vi "Untitled 7 (SubVI).vi"(8 "y 2":i32, 9 "x 2":i32, 10 "y 1":i32, 11 "x 1":i32) -> (1 "Boolean":bool, 2 "Array":cluster{"x 1":i32, i32}[](array[cluster]))   [LabVIEW 2017]
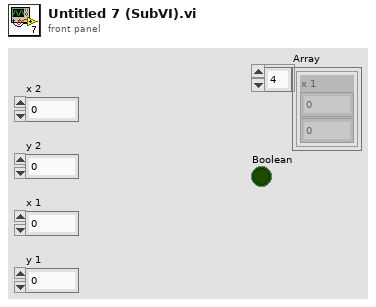
[diagram p1: front panel]
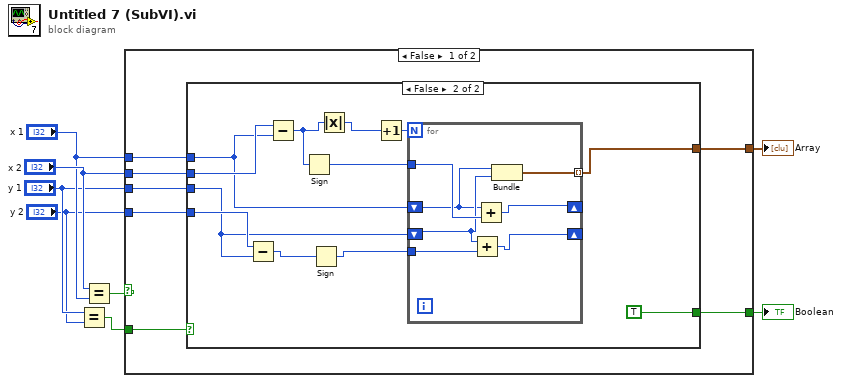
[diagram p0: block diagram]
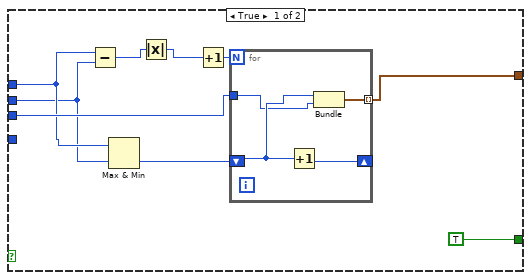
[diagram p2: hidden frame]
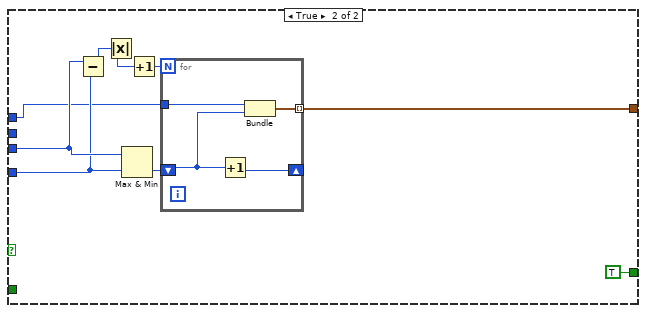
[diagram p3: hidden frame]
diagram:
  n1 = Equal?(x="y 1", y="y 2") -> (x = y?=w7:bool)
  n2 = Equal?(x="x 2", y="x 1") -> (x = y?=w8:bool)
  n3 = case shown="False" w8 {
    tunnel: w7 -> [w15 _]
    tunnel: "x 2" -> [w14 _]
    tunnel: "x 1" -> [w13 w52]
    tunnel: "y 1" -> [w12 w55]
    tunnel: "y 2" -> [w11 w54]
    tunnel: [w10 w51] -> w2
    tunnel: [w9 TRUE] -> w1
    frame False {
      n4 = case shown="False" w15 {
        tunnel: w14 -> [w19 w38]
        tunnel: w13 -> [w20 w35]
        tunnel: w12 -> [w21 w29]
        tunnel: w11 -> [_ w32]
        tunnel: [w22 w39] -> w10
        tunnel: [TRUE TRUE] -> w9
        frame True {
          n5 = Subtract(x=w20, y=w19) -> (x-y=w18:i32)
          n6 = Max & Min(x=w20, y=w19) -> (min(x,y)=w23:i32)  [unwired: 1 out]
          n7 = Absolute Value(x=w18) -> (abs(x)=w17:i32)
          n8 = Increment(x=w17) -> (x+1=w24:i32)
          n9 = for {
            N: w24 -> [_]
            shift-right: [w28] -> _
            shift-left: w23 -> [w26]
            tunnel: w21 -> [w25]
            tunnel: [w27] -> w22 mode=indexing
            n10 = Increment(x=w26) -> (x+1=w28:i32)
            n11 = Bundle(w26, "y 1"=w25) -> (w27:cluster{i32, "y 1":i32})  [unwired: 1 in]
          }
        }
        frame False {
          n12 = Subtract(x=w32, y=w29) -> (x-y=w31:i32)
          n13 = Subtract(x=w38, y=w35) -> (x-y=w34:i32)
          n14 = Sign(1:w34) -> (0:w33:i32)
          n15 = Sign(1:w31) -> (0:w30:i32)
          n16 = Absolute Value(x=w34) -> (abs(x)=w37:i32)
          n17 = Increment(x=w37) -> (x+1=w40:i32)
          n18 = for {
            N: w40 -> [_]
            shift-right: [w45] -> _
            shift-left: w29 -> [w42]
            tunnel: [w47] -> w39 mode=indexing
            shift-right: [w46] -> _
            shift-left: w35 -> [w41]
            tunnel: w33 -> [w44]
            tunnel: w30 -> [w43]
            n19 = Add(x=w42, y=w43) -> (x+y=w45:i32)
            n20 = Add(x=w41, y=w44) -> (x+y=w46:i32)
            n21 = Bundle("x 1"=w41, "y 1"=w42) -> (w47:cluster{"x 1":i32, "y 1":i32})  [unwired: 1 in]
          }
        }
      }
    }
    frame True {
      n22 = Subtract(x=w55, y=w54) -> (x-y=w49:i32)
      n23 = Absolute Value(x=w49) -> (abs(x)=w50:i32)
      n24 = Max & Min(x=w55, y=w54) -> (min(x,y)=w53:i32)  [unwired: 1 out]
      n25 = Increment(x=w50) -> (x+1=w56:i32)
      n26 = for {
        N: w56 -> [_]
        shift-right: [w60] -> _
        shift-left: w53 -> [w58]
        tunnel: w52 -> [w59]
        tunnel: [w57] -> w51 mode=indexing
        n27 = Increment(x=w58) -> (x+1=w60:i32)
        n28 = Bundle("x 1"=w59, w58) -> (w57:cluster{"x 1":i32, i32})  [unwired: 1 in]
      }
    }
  }
  "Array" <- w2
  "Boolean" <- w1
